vi "Initialize.vi"(8 "error in (no error)":errorcluster, 10 "Handle":T1 format="%x", 11 "Node in":refnum<class "ThermotronDriver.lvclass"> caption="Timed Node in") -> (0 "error out":errorcluster, 3 "Node out":refnum<class "ThermotronDriver.lvclass"> caption="Timed Node out")   [LabVIEW 2023, in "ThermotronDriver.lvlib" / "ThermotronDriver.lvclass"]
uses:
  ThermotronDriver.lvclass
  ThermotronDriver.lvclass/ThermotronDriver.ctl
  <vilib>/ADAS Replay HIL/AdasHilServices/AdasHilChannelServices.lvlib
  <vilib>/ADAS Replay HIL/AdasHilServices/Server Mode.ctl
  <vilib>/ADAS Replay HIL/Template Node/Plugin/Template Node/Template Node.lvclass
  Program Files/National Instruments/ADAS Replay HIL/EVO SDK/Linux RT/evoLabVIEWAPI/evoPluginSDK.lvlibp/VIs/TypeDefs/Handle.ctl
  Program Files/National Instruments/ADAS Replay HIL/EVO SDK/Linux RT/evoLabVIEWAPI/evoPluginSDK.lvlibp
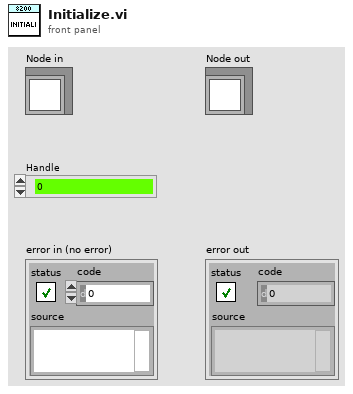
[diagram p1: front panel]
types:
  T1 = typedef "evoPluginSDK.lvlibp/Handle.ctl" = u64
  T2 = typedef "AdasHilChannelServices.lvlib/Server Mode.ctl" = enum8{"External Process", "In Process"}
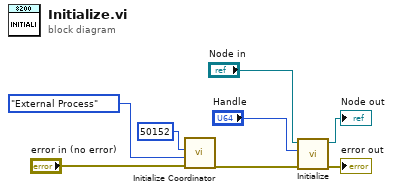
[diagram p0: block diagram]
diagram:
  n1 = call <vilib>:"Initialize Coordinator.vi"("error in"="error in (no error)", "Server Port"=50152, "Server Mode"=Server_Mode."External Process") -> ("error out"=w3:errorcluster)  [unwired: 8 in]
  n2 = call-parent "Initialize.vi"("error in (no error)"=w3, "Handle"="Handle", "Node in"="Node in") -> ("error out"=→"error out":errorcluster, "Node out"=→"Node out":refnum<class "ThermotronDriver.lvclass">)  [unwired: 7 in]
